vi "实时数据指令打包.vi"(8 "错误 i":errorcluster caption="错误常量", 11 "测量值":dbl=0.1 format="%#_13g") -> (0 "错误 o":errorcluster caption="错误常量", 3 "完整输出":string)   [LabVIEW 2017]
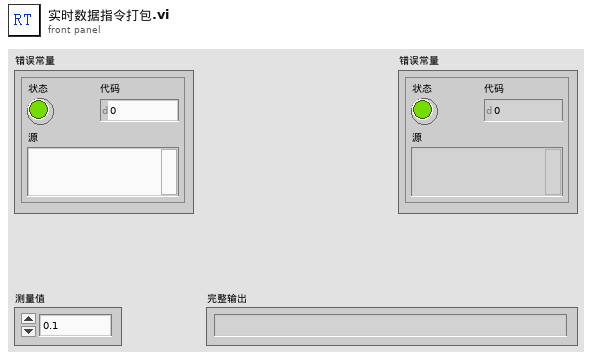
[diagram p1: front panel]
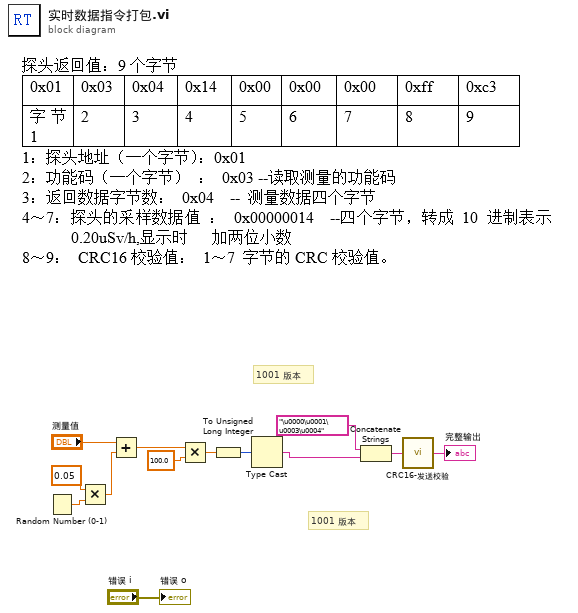
[diagram p0: block diagram]
diagram:
  # "1001 版本"
  # "1001 版本"
  n1 = Random Number (0-1)() -> (number: 0 to 1=w5:dbl)
  n2 = Multiply(x=0.05, y=w5) -> (x*y=w7:dbl)
  n3 = Add(x="测量值", y=w7) -> (x+y=w8:dbl)
  n4 = Multiply(x=w8, y=100.0) -> (x*y=w10:dbl)
  n5 = To Unsigned Long Integer(number=w10) -> (unsigned 32bit integer=w11:u32)
  n6 = Type Cast(x=w11) -> (*(type *) &x=w12:string)  [unwired: 1 in]
  n7 = Concatenate Strings("\u0000\u0001\u0003\u0004" ("字符串"), w12) -> (w13:string)
  n8 = call "CRC16-发送校验.vi"("净数据"=w13) -> ("完整输出"=→"完整输出":string)
  "错误 o" <- "错误 i"
